vi "Coerce Z Output Waveform.vi"(1 "X Output Waveform":waveform(dbl)) -> (0 "Coerced X Output Waveform":waveform(dbl))   [LabVIEW 2013]
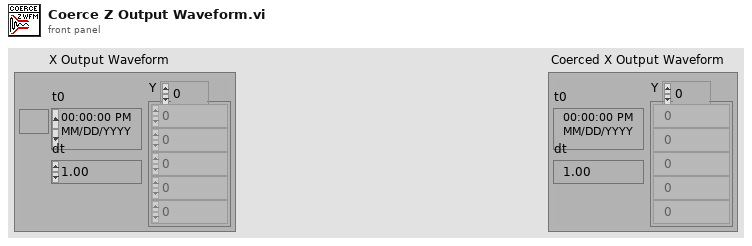
[diagram p1: front panel]
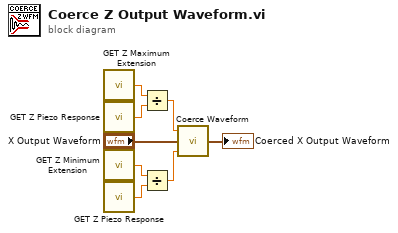
[diagram p0: block diagram]
diagram:
  n1 = call "GET Z Maximum Extension.vi"() -> ("Z Maximum Extension"=w6:dbl)
  n2 = call "GET Z Piezo Response.vi"() -> ("Z Piezo Response"=w5:dbl)
  n3 = call "GET Z Minimum Extension.vi"() -> ("Z Minimum Extension"=w4:dbl)
  n4 = call "GET Z Piezo Response.vi"() -> ("Z Piezo Response"=w3:dbl)
  n5 = Divide(x=w6, y=w5) -> (x/y=w1:dbl)
  n6 = Divide(x=w4, y=w3) -> (x/y=w2:dbl)
  n7 = call "Coerce Waveform.vi"("Lower Limit"=w2, "Output Waveform"="X Output Waveform", "Upper Limit"=w1) -> ("Coerced Output Waveform"=→"Coerced X Output Waveform":waveform(dbl))
